vi "Write Slices.vi"(8 "error in (no error)":errorcluster, 10 "Slices[]":T1[](array[typedef]), 11 "PieChart in":refnum<class "PieChart.lvclass">) -> (0 "error out":errorcluster, 3 "PieChart out":refnum<class "PieChart.lvclass">)   [LabVIEW 2018, in "PieChart.lvclass"]
uses:
  PieChart.lvclass
  Pie Slice.ctl
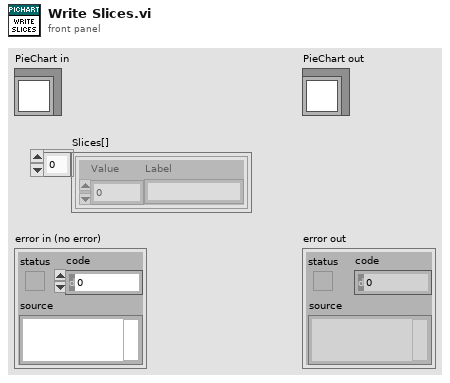
[diagram p1: front panel]
types:
  T1 = typedef "PieChart.lvclass/Pie Slice.ctl" = cluster{"Value":dbl, "Label":string}
  T2 = typedef "PieChart.lvclass/State Data.ctl" = cluster{"Title":string, "Values[]":dbl[], "Labels[]":string[], "Colors[]":u32[], "Include Legend?":bool, "Include Title?":bool, "Title Font":T3, "Legend Font":T3, "Selection":i32, "Slice Positions":T4}
  T3 = typedef "LVFontTypeDef.ctl" = cluster{"Font Name":string, "Size":u16, "Bold":bool, "Italic":bool, "Underline":bool, "Strikeout":bool, "Color":u32}
  T4 = typedef "PieChart.lvclass/Pie info for Click.ctl" = cluster{"Slice Positions":cluster{"Start":i16, "End":i16}[], "Center Position":T5, "Radius":i16}
  T5 = typedef "LVBoundsTypeDef.ctl" = cluster{"Width":u32, "Height":u32}
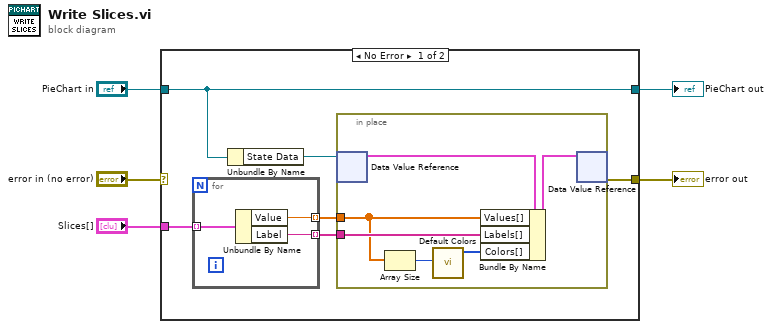
[diagram p0: block diagram]
diagram:
  n1 = case shown="No Error" "error in (no error)" {
    selector: "error in (no error)" -> [_ w22]
    tunnel: [w9 w22] -> w4
    tunnel: [w10 w21] -> w2
    tunnel: "PieChart in" -> [w10 w21]
    tunnel: "Slices[]" -> [w8 _]
    frame No Error {
      n2 = for {
        tunnel: w8 -> [w14] mode=indexing
        tunnel: [w13] -> w7 mode=indexing
        tunnel: [w12] -> w6 mode=indexing
        n3 = Unbundle By Name(w14) -> ("Value"=w13:dbl, "Label"=w12:string)
      }
      n4 = Unbundle By Name(w10) -> ("State Data"=w11:refnum<data-value>)
      n5 = in-place {
        in-place-border: w7 -> [w16]
        in-place-border: w6 -> [w18]
        n6 = in-place-dvr #1(w11) -> (w20:T2)  [unwired: 1 out]
        n7 = Array Size(array=w16) -> (size(s)=w15:i32)
        n8 = call "Default Colors.vi"("Number of Entries"=w15) -> ("Colors[] out"=w17:u32[])  [unwired: 10 in]
        n9 = Bundle By Name(cluster=w20, "Values[]"=w16, "Labels[]"=w18, "Colors[]"=w17) -> (w19:T2)
        n10 = in-place-dvr #1(w19) -> (w9:errorcluster)  [unwired: 1 out]
      }
    }
    frame Error {
    }
  }
  "error out" <- w4
  "PieChart out" <- w2
